vi "GlobalConfig.vi"() -> ()   [LabVIEW 2014]
panel:
  in  "ConfigFile":path
  # "Getting a little recursive here :-)"
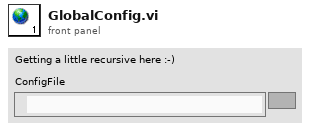
[diagram p1: front panel]
diagram:
